vi "IOCtestRcv.vi"() -> ()   [LabVIEW 2018]
uses:
  <userlib>/caLab/Private/Get_PV.vi
panel:
  out "Waveform Chart 2":dbl(graph)
  out "Status":bool
  out "Waveform Chart":dbl(graph)
  out "1rst Value (number)":dbl
  in  "stop":bool
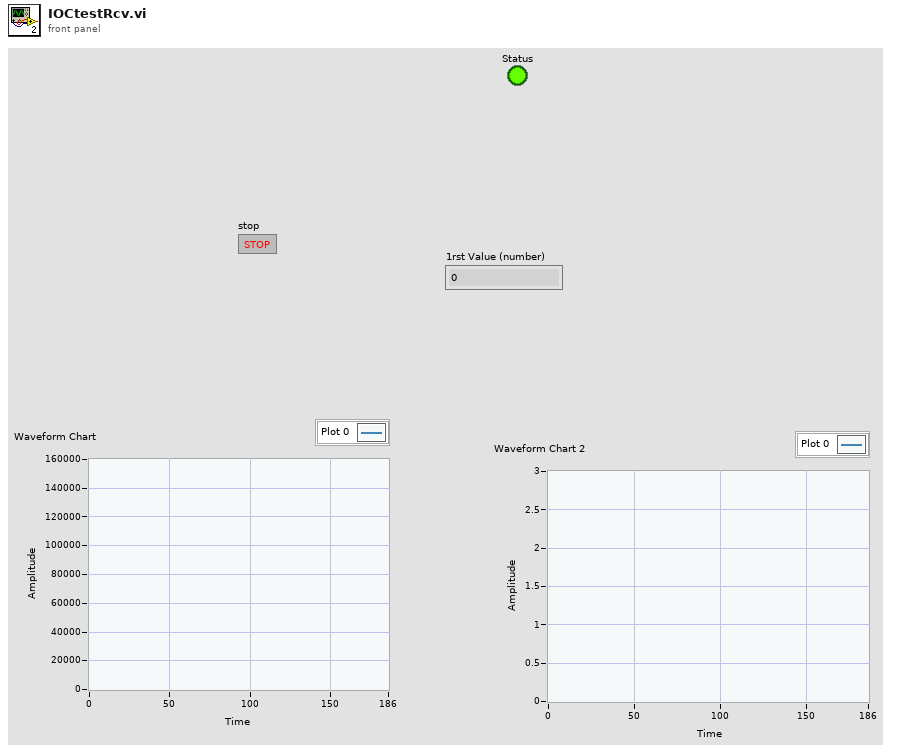
[diagram p1: front panel]
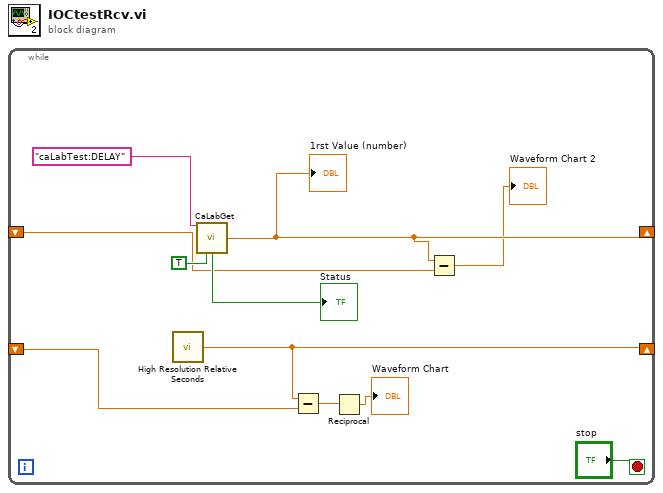
[diagram p0: block diagram]
diagram:
  n1 = while {
    shift-right: [w8] -> _
    shift-left: _ -> [w7]
    shift-right: [w3] -> _
    shift-left: _ -> [w2]
    stop <- "stop" stop-if-true
    n2 = call <vilib>:"High Resolution Relative Seconds.vi"() -> ("relative seconds"=w8:dbl)
    n3 = call-poly <userlib>:"CaLabGet.vi"("PV Name"="caLabTest:DELAY", "NoMDEL(F)"=TRUE) -> ("1rst Value (number)"=w3:dbl, "Status"=→"Status":bool)  [unwired: 7 in, 5 out]
    "1rst Value (number)" <- w3
    n4 = Subtract(x=w8, y=w7) -> (x-y=w9:dbl)
    n5 = Reciprocal(x=w9) -> (1/x=→"Waveform Chart":dbl)
    n6 = Subtract(x=w3, y=w2) -> (x-y=→"Waveform Chart 2":dbl)
  }
